vi "ADI_IMU_ADIS16470_Open.vi"(5 "Calibrate On Open":bool=TRUE, 7 "Calibration Time (s)":dbl=3.0, 8 "error in":errorcluster, 10 "Yaw Axis":enum16{"X", "Y", "Z"}(ring)=enum."Z", 11 "SPI Chip Select":T2=enum."SPI MXP") -> (0 "error out":errorcluster, 2 "Offset Compensated Data Out":dbl[](array[numeric]), 3 "ADI IMU DevRef Out":T1={"DevStatus"={"status"=FALSE, "code"=0, "source"=""}, "Handle"=0, "SPI Bus"=enum."SPI On-Board, CS0", "Device Found"=FALSE, "Device Ready"=FALSE, "Yaw Axis"=enum."Z", "Serial"=0, "Bytes Per Sample"=0, "Calibrate On Open?"=FALSE})   [LabVIEW 2017, in "ADIS16470_IMU.lvlib"]
doc: "Initiates communication between an Analog Devices MXP IMU and the RoboRIO."
uses:
  ADIS16470_IMU.lvlib
  <vilib>/Rock Robotics/SystemInterfaces/spilib/spi_bus.ctl
  ADI_IMU_ADIS16470_IMUDevRef.ctl
  <vilib>/Rock Robotics/WPI/SPI/WPI_SPIMode.ctl
  <vilib>/Rock Robotics/SystemInterfaces/DIO/FPGA_DIOChannel.ctl
  ADI_IMU_ADIS16470_Registers.ctl
  <vilib>/Rock Robotics/SystemInterfaces/NetworkCommunication/NetComm_UsageReport_ResourceType.ctl
  <vilib>/Rock Robotics/WPI/Counter/WPI_CounterDigitalInputToDigitalSource.vi
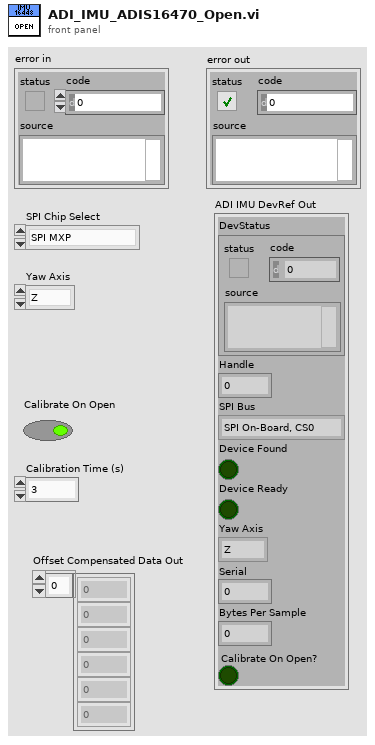
[diagram p1: front panel]
types:
  T1 = typedef "ADIS16470_IMU.lvlib/ADI_IMU_ADIS16470_IMUDevRef.ctl" = cluster{"DevStatus":errorcluster, "Handle":i32, "SPI Bus":T2, "Device Found":bool, "Device Ready":bool, "Yaw Axis":enum16{"X", "Y", "Z"}, "Serial":u16, "Bytes Per Sample":u16, "Calibrate On Open?":bool}
  T2 = typedef "spi_bus.ctl" = enum16{"SPI On-Board, CS0", "SPI On-Board, CS1", "SPI On-Board, CS2", "SPI On-Board, CS3", "SPI MXP", "Invalid"}
  T3 = typedef "FPGA_DIOChannel.ctl" = enum8{"DIO 0", "DIO 1", "DIO 2", "DIO 3", "DIO 4", "DIO 5", "DIO 6", "DIO 7", "DIO 8", "DIO 9", "DIO MXP 0", "DIO MXP 1", "DIO MXP 2", "DIO MXP 3", "DIO MXP 4", "DIO MXP 5", "DIO MXP 6", "DIO MXP 7", "DIO MXP 8", "DIO MXP 9", "DIO MXP 10", "DIO MXP 11", "DIO MXP 12", "DIO MXP 13", "DIO MXP 14", "DIO MXP 15", "SPI Port CS1", "SPI Port CS2", "SPI Port CS3", "SPI Port MISO", "SPI Port MOSI", "Invalid"}
  T4 = typedef "WPI_SPIMode.ctl" = enum16{"Mode 0 (Clk Idle Low,Sample on Leading)", "Mode 1 (Clk Idle Low,Sample on Trailing)", "Mode 2 (Clk Idle High,Sample on Leading)", "Mode 3 (Clk Idle High,Sample on Trailing)"}
  T5 = typedef "NetComm_UsageReport_ResourceType.ctl" = enum8{"Controller", "Module", "Language", "CANPlugin", "Accelerometer", "ADXL345", "AnalogChannel", "AnalogTrigger", "AnalogTriggerOutput", "CANJaguar", "Compressor", "Counter", "Dashboard", "DigitalInput", "DigitalOutput", "DriverStationCIO", "DriverStationEIO", "DriverStationLCD", "Encoder", "GearTooth", "Gyro", "I2C", "Framework", "Jaguar", "Joystick", "Kinect", "KinectStick", "PIDController", "Preferences", "PWM", "Relay", "RobotDrive", "SerialPort", "Servo", "Solenoid", "SPI", "Task", "Ultrasonic", "Victor", "Button", "Command", "AxisCamera", "PCVideoServer", "SmartDashboard", "Talon", "HiTechnicColorSensor", "HiTechnicAccel", "HiTechnicCompass", "SRF08", "AnalogOutput", "Victor SP", "Talon SRX", "CAN Talon SRX", "ADXL362 Accel", "ADXRS450 Gyro", "Rev SPARK", "Mindsensors SD540", "Digital Filter", "ADIS16448", "PDP", "PCM", "PigeonIMU", "Nidec Brushless", "CTRE CANifier", "CTRE Future 0", "CTRE Future 1", "CTRE Future 2", "CTRE Future 3", "CTRE Future 4", "CTRE Future 5", "CTRE Future 6"}
  T6 = typedef "ADIS16470_IMU.lvlib/ADI_IMU_ADIS16470_Registers.ctl" = u8
  T7 = typedef "WPI_DigitalOutputDevRef.ctl" = cluster{"DIO Channel":T3, "DevStatus":errorcluster}
  T8 = typedef "WPI_DigitalInputDevRef.ctl" = cluster{"DevStatus":errorcluster, "DIO Channel":T3}
  T9 = typedef "WPI_SPIDevRef.ctl" = cluster{"DevStatus":errorcluster, "Handle":i32, "SPI Bus":T2}
  T10 = typedef "FPGA_CounterEncoderSourceConvertionLVSourceType.ctl" = cluster{"DevStatus":errorcluster, "AnalogTriggerMode?":bool, "DigitalMode":cluster{"DIO Channel":T11}, "AnalogTriggerMode":cluster{"AnalogTriggerIndex":T12, "OutputType":T13}}
  T11 = typedef "FPGA_DIODigitalSourceChannel.ctl" = enum8{"DIO 0", "DIO 1", "DIO 2", "DIO 3", "DIO 4", "DIO 5", "DIO 6", "DIO 7", "DIO 8", "DIO 9", "DIO MXP 0", "DIO MXP 1", "DIO MXP 2", "DIO MXP 3", "DIO MXP 4", "DIO MXP 5", "DIO MXP 6", "DIO MXP 7", "DIO MXP 8", "DIO MXP 9", "DIO MXP 10", "DIO MXP 11", "DIO MXP 12", "DIO MXP 13", "DIO MXP 14", "DIO MXP 15", "SPI Port CS1", "SPI Port CS2", "SPI Port CS3", "SPI Port MISO", "SPI Port MOSI", "Disabled"}
  T12 = typedef "FPGA_AnalogTriggerIndex.ctl" = enum8{"Trig 0", "Trig 1", "Trig 2", "Trig 3", "Trig 4", "Trig 5", "Trig 6", "Trig 7", "Invalid"}
  T13 = typedef "FPGA_AnalogTriggerOutType.ctl" = enum16{"InWindow", "TriggerState", "Rising", "Falling"}
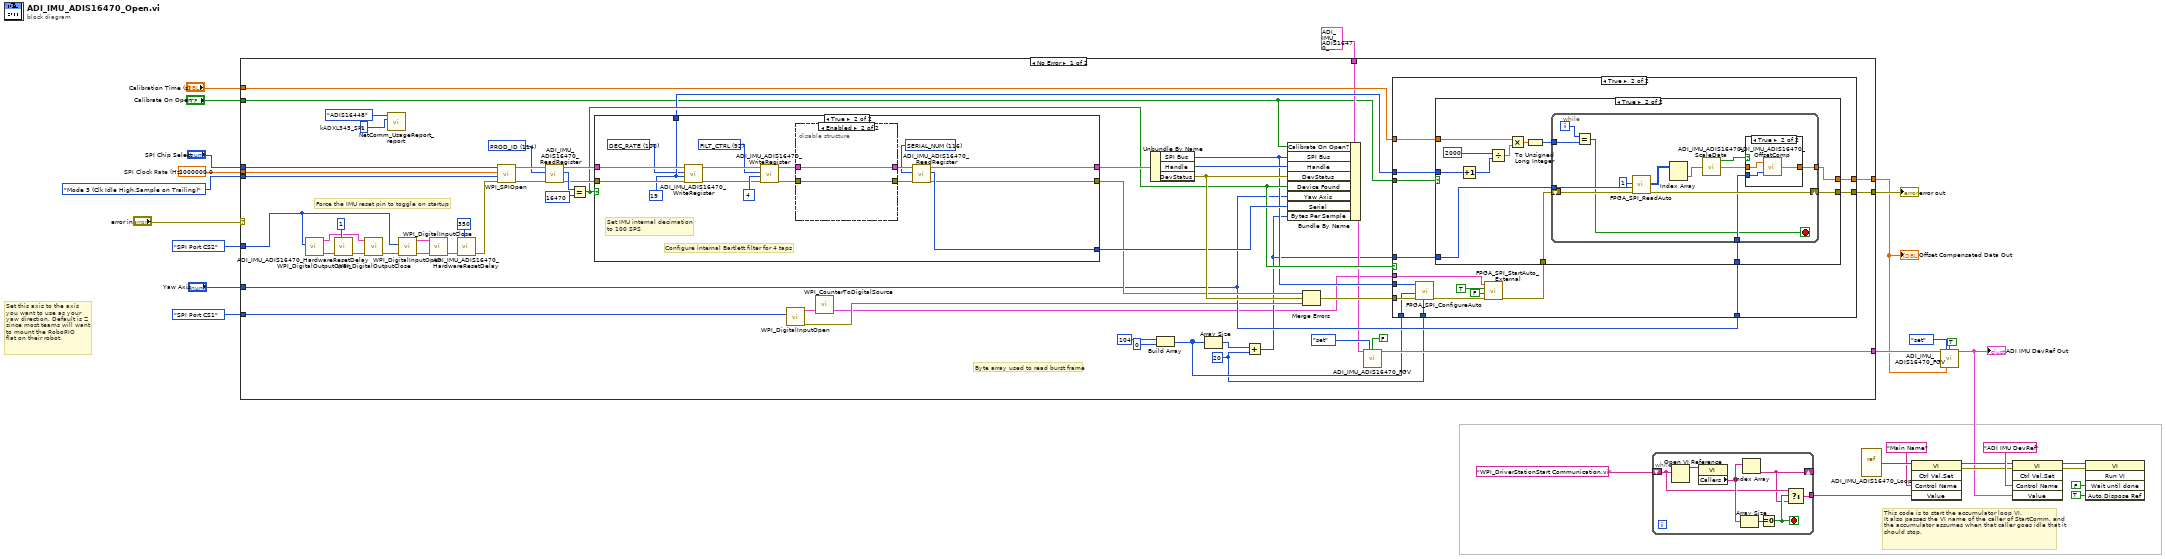
[diagram p0: block diagram]
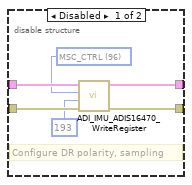
[diagram p6: hidden frame]
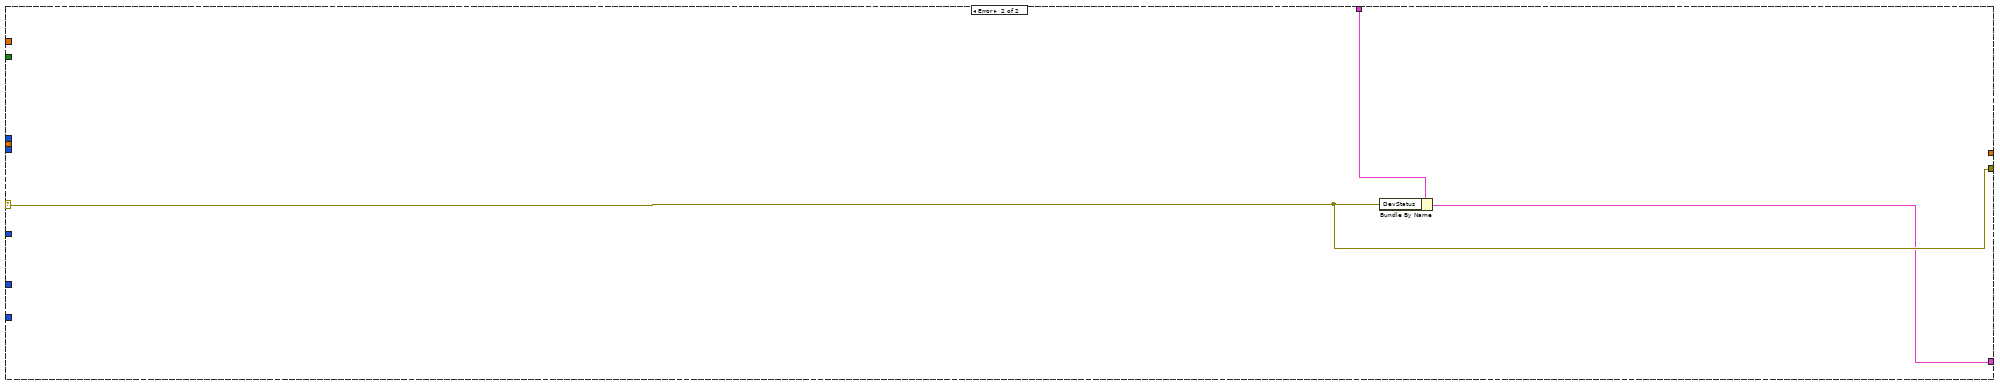
[diagram p7: hidden frame]
diagram:
  w27 = 1000000.0  # SPI Clock Rate (Hz)
  # "This code is to start the accumulator loop VI.\nIt also passes the VI name of the caller of StartComm, and the accumulator assumes when that caller goes idle that it should stop."
  # "Set this axis to the axis\nyou want to use as your\nyaw direction. Default is Z\nsince most teams will want \nto mount the RoboRIO\nflat on their robot."
  n1 = case shown="No Error" "error in" {
    selector: "error in" -> [_ w154]
    tunnel: w27 -> [w79 _]
    tunnel: WPI_SPIMode."Mode 3 (Clk Idle High,Sample on Trailing)" ("Mode (3)") -> [w78 _]
    tunnel: "SPI Chip Select" -> [w77 _]
    tunnel: FPGA_DIOChannel."SPI Port CS1" ("DIO Channel") -> [w57 _]
    tunnel: "Yaw Axis" -> [w54 _]
    tunnel: FPGA_DIOChannel."SPI Port CS2" ("DIO Channel") -> [w76 _]
    tunnel: "Calibrate On Open" -> [w33 _]
    tunnel: "Calibration Time (s)" -> [w55 _]
    tunnel: T1 {"DevStatus"={"status"=FALSE, "code"=0, "source"=""}, "Handle"=0, "SPI Bus"=enum."SPI On-Board, CS0", "Device Found"=FALSE, "Device Ready"=FALSE, "Yaw Axis"=enum."Z", "Serial"=0, "Bytes Per Sample"=0, "Calibrate On Open?"=FALSE} ("SimpleGyroDevRef 2") -> [w53 w155]
    tunnel: [w52 w154] -> w6
    tunnel: [w48 w153] -> w3
    tunnel: [w47 _] -> w2
    frame No Error {
      w30 = 20 ("dimension size")
      w71 = u8 1  # kADXL345_SPI
      w67 = T6 114 items=["DIAG_STAT"=2, "X_GYRO"=6, "Y_GYRO"=10, "Z_GYRO"=14, "X_ACCEL"=18, "Y_ACCEL"=22, "Z_ACCEL"=26, "TEMP"=28, "TIME_STAMP"=30, "FILT_CTRL"=92, "MSC_CTRL"=96, "DEC_RATE"=100, "NULL_CFG"=102, "GLOB_CMD"=104, "PROD_ID"=114, "SERIAL_NUM"=116] ("ADIS16448 Register")
      # "Byte array used to read burst frame"
      # "Force the IMU reset pin to toggle on startup"
      n2 = call <vilib>:"WPI_DigitalOutputOpen.vi"("DIO Channel"=w76) -> ("error out"=w44:errorcluster, "DigitalOutputDevRef"=w38:T7)  [unwired: 9 in]
      n3 = call "ADI_IMU_ADIS16470_HardwareResetDelay.vi"("Delay (ms)"=u32 1, "error in"=w44) -> ("error out"=w45:errorcluster)  [unwired: 9 in]
      n4 = call <vilib>:"WPI_DigitalOutputClose.vi"("error in (no error)"=w45, "DigitalOutputDevRef"=w38) -> ("error out"=w43:errorcluster)  [unwired: 9 in]
      n5 = call <vilib>:"NetComm_UsageReport_report.vi"("Instance Number"=w71, "Resource Type"=NetComm_UsageReport_ResourceType."ADIS16448") -> ()  [unwired: 10 in]
      n6 = call <vilib>:"WPI_DigitalInputOpen.vi"("error in (no error)"=w43, "DIO Channel"=w76) -> ("error out"=w42:errorcluster, "DigitalInputDevRef"=w41:T8)  [unwired: 8 in]
      n7 = call <vilib>:"WPI_DigitalInputClose.vi"("error in (no error)"=w42, "DigitalInputDevRef"=w41) -> ("error out"=w40:errorcluster)  [unwired: 9 in]
      n8 = call "ADI_IMU_ADIS16470_HardwareResetDelay.vi"("Delay (ms)"=u32 350, "error in"=w40) -> ("error out"=w72:errorcluster)  [unwired: 9 in]
      n9 = call <vilib>:"WPI_SPIOpen.vi"("error in"=w72, "Mode (3)"=w78, "Clock Rate (Hz)"=w79, "SPI Bus"=w77) -> ("error out"=w68:errorcluster, "SPIDevRef"=w69:T9)  [unwired: 6 in]
      n10 = call "ADI_IMU_ADIS16470_ReadRegister.vi"("error in (no error)"=w68, "ADIS16448 Register"=w67, "SPIDevRef in"=w69) -> ("error out"=w63:errorcluster, "Register Value"=w66:u16, "SPIDevRef out"=w64:T9)  [unwired: 6 in]
      n11 = Equal?(x=w66, y=u16 16470) -> (x = y?=w59:bool)
      n12 = case shown="True" w59 {
        tunnel: [_ w143] -> w73
        tunnel: [w128 w130] -> w62
        tunnel: [w127 w129] -> w61
        tunnel: w64 -> [w128 w136]
        tunnel: w63 -> [w127 w135]
        tunnel: [_ w134] -> w56
        frame False {
        }
        frame True {
          w131 = T6 116 items=["DIAG_STAT"=2, "X_GYRO"=6, "Y_GYRO"=10, "Z_GYRO"=14, "X_ACCEL"=18, "Y_ACCEL"=22, "Z_ACCEL"=26, "TEMP"=28, "TIME_STAMP"=30, "FILT_CTRL"=92, "MSC_CTRL"=96, "DEC_RATE"=100, "NULL_CFG"=102, "GLOB_CMD"=104, "PROD_ID"=114, "SERIAL_NUM"=116] ("ADIS16448 Register")
          w132 = T6 92 items=["DIAG_STAT"=2, "X_GYRO"=6, "Y_GYRO"=10, "Z_GYRO"=14, "X_ACCEL"=18, "Y_ACCEL"=22, "Z_ACCEL"=26, "TEMP"=28, "TIME_STAMP"=30, "FILT_CTRL"=92, "MSC_CTRL"=96, "DEC_RATE"=100, "NULL_CFG"=102, "GLOB_CMD"=104, "PROD_ID"=114, "SERIAL_NUM"=116] ("ADIS16448 Register")
          w133 = T6 100 items=["DIAG_STAT"=2, "X_GYRO"=6, "Y_GYRO"=10, "Z_GYRO"=14, "X_ACCEL"=18, "Y_ACCEL"=22, "Z_ACCEL"=26, "TEMP"=28, "TIME_STAMP"=30, "FILT_CTRL"=92, "MSC_CTRL"=96, "DEC_RATE"=100, "NULL_CFG"=102, "GLOB_CMD"=104, "PROD_ID"=114, "SERIAL_NUM"=116] ("ADIS16448 Register")
          w134 = u16 19 ("Data")
          # "Configure internal Bartlett filter for 4 taps"
          # "Set IMU internal decimation\nto 100 SPS"
          n13 = call "ADI_IMU_ADIS16470_WriteRegister.vi"("error in (no error)"=w135, "Data"=w134, "ADIS16448 Register"=w133, "SPIDevRef in"=w136) -> ("error out"=w141:errorcluster, "SPIDevRef out"=w142:T9)  [unwired: 6 in]
          n14 = call "ADI_IMU_ADIS16470_WriteRegister.vi"("error in (no error)"=w141, "Data"=u16 4, "ADIS16448 Register"=w132, "SPIDevRef in"=w142) -> ("error out"=w139:errorcluster, "SPIDevRef out"=w140:T9)  [unwired: 6 in]
          n15 = disable-structure shown="Enabled" {
            disable-tunnel: w140 -> [w150 w152]
            disable-tunnel: w139 -> [w149 w151]
            disable-tunnel: [w148 w152] -> w138
            disable-tunnel: [w147 w151] -> w137
            frame Disabled {
              w145 = T6 96 items=["DIAG_STAT"=2, "X_GYRO"=6, "Y_GYRO"=10, "Z_GYRO"=14, "X_ACCEL"=18, "Y_ACCEL"=22, "Z_ACCEL"=26, "TEMP"=28, "TIME_STAMP"=30, "FILT_CTRL"=92, "MSC_CTRL"=96, "DEC_RATE"=100, "NULL_CFG"=102, "GLOB_CMD"=104, "PROD_ID"=114, "SERIAL_NUM"=116] ("ADIS16448 Register")
              # "Configure DR polarity, sampling"
              n16 = call "ADI_IMU_ADIS16470_WriteRegister.vi"("error in (no error)"=w149, "Data"=u16 193, "ADIS16448 Register"=w145, "SPIDevRef in"=w150) -> ("error out"=w147:errorcluster, "SPIDevRef out"=w148:T9)  [unwired: 6 in]
            }
            frame Enabled {
            }
          }
          n17 = call "ADI_IMU_ADIS16470_ReadRegister.vi"("error in (no error)"=w137, "ADIS16448 Register"=w131, "SPIDevRef in"=w138) -> ("error out"=w129:errorcluster, "Register Value"=w143:u16, "SPIDevRef out"=w130:T9)  [unwired: 6 in]
        }
      }
      n18 = call <vilib>:"WPI_DigitalInputOpen.vi"("DIO Channel"=w57) -> ("error out"=w37:errorcluster, "DigitalInputDevRef"=w28:T8)  [unwired: 9 in]
      n19 = call-poly <vilib>:"WPI_CounterToDigitalSource.vi"("DigitalInputDevRef"=w28) -> ("Digital Source"=w29:T10)  [unwired: 6 in]
      n20 = Unbundle By Name(w62) -> ("SPI Bus"=w58:T2, "Handle"=w75:i32, "DevStatus"=w74:errorcluster)
      n21 = Build Array(u8 104 ("hi"), u8 0 ("element")) -> (w34:u8[])
      n22 = Array Size(array=w34) -> (size(s)=w32:i32)
      n23 = Add(x=w32, y=w30) -> (x+y=w31:i32)
      n24 = Bundle By Name(cluster=w53, "Calibrate On Open?"=w33, "SPI Bus"=w58, "Handle"=w75, "DevStatus"=w74, "Device Found"=w59, "Yaw Axis"=w54, "Serial"=w73, "Bytes Per Sample"=w31) -> (w49:T1)
      n25 = Merge Errors(w61, w74, w37) -> (w60:errorcluster)
      n26 = call "ADI_IMU_ADIS16470_FGV.vi"("ADI IMU DevRef"=w49, "Operation"=enum16{"set", "get", "set reset"}."set", "Sensor Ready?"=FALSE) -> ("ADI IMU DevRef Out"=w48:T1)  [unwired: 7 in, 5 out]
      n27 = case shown="True" w59 {
        tunnel: w60 -> [w80 w96]
        tunnel: w58 -> [_ w95]
        tunnel: w34 -> [_ w83]
        tunnel: w29 -> [_ w91]
        tunnel: w33 -> [_ w90]
        tunnel: w56 -> [_ w88]
        tunnel: w55 -> [_ w87]
        tunnel: [_ w86] -> w47
        tunnel: w54 -> [_ w85]
        tunnel: [w80 w84] -> w52
        tunnel: w31 -> [_ w82]
        tunnel: w30 -> [_ w81]
        frame False {
        }
        frame True {
          n28 = call <vilib>:"FPGA_SPI_ConfigureAuto.vi"("SPI Auto Zero Byte Count"=w81, "error in"=w96, "SPI Auto TX Byte Array"=w83, "SPI Bus"=w95) -> ("error out"=w94:errorcluster)  [unwired: 7 in]
          n29 = call <vilib>:"FPGA_SPI_StartAuto_External.vi"("error in (no error)"=w94, "Falling Edge"=FALSE, "Rising Edge"=TRUE, "Source"=w91) -> ("error out"=w89:errorcluster)  [unwired: 7 in]
          n30 = case shown="True" w90 {
            tunnel: w89 -> [w97 w109]
            tunnel: w88 -> [_ w99]
            tunnel: w87 -> [_ w106]
            tunnel: [_ w104] -> w86
            tunnel: w85 -> [_ w105]
            tunnel: [w97 w103] -> w84
            tunnel: w82 -> [_ w101]
            frame False {
            }
            frame True {
              n31 = Increment(x=w99) -> (x+1=w98:u16)
              n32 = Divide(x=2000, y=w98) -> (x/y=w108:dbl)
              n33 = Multiply(x=w106, y=w108) -> (x*y=w107:dbl)
              n34 = To Unsigned Long Integer(number=w107) -> (unsigned 32bit integer=w102:u32)
              n35 = while {
                shift-right: [w121] -> w103
                shift-left: w109 -> [w122]
                tunnel: w105 -> [w120]
                tunnel: [w119] -> w104
                tunnel: w101 -> [w117]
                tunnel: w102 -> [w114]
                i -> [w115]
                stop <- w113 stop-if-true
                n36 = Equal?(x=w115, y=w114) -> (x = y?=w113:bool)
                n37 = call <vilib>:"FPGA_SPI_ReadAuto.vi"("error in (no error)"=w122, "Bytes per Sample"=w117, "Samples to Read"=u32 1) -> ("error out"=w121:errorcluster, "Data"=w112:u8[][])  [unwired: 7 in]
                n38 = Index Array(array=w112) -> (element=w111:u8[])  [unwired: 2 in]
                n39 = call "ADI_IMU_ADIS16470_ScaleData.vi"("Received Data"=w111) -> ("Data Array"=w118:dbl[], "Data Good?"=w110:bool)  [unwired: 3 in]
                n40 = case shown="True" w110 {
                  tunnel: w120 -> [_ w126]
                  tunnel: [w123 w125] -> w119
                  tunnel: w118 -> [w123 w124]
                  frame False {
                  }
                  frame True {
                    n41 = call "ADI_IMU_ADIS16470_OffsetComp.vi"("Yaw Axis"=w126, "Raw Data"=w124) -> ("Offset Compensated Data"=w125:dbl[])
                  }
                }
              }
            }
          }
        }
      }
    }
    frame Error {
      n42 = Bundle By Name(cluster=w155, "DevStatus"=w154) -> (w153:T1)
    }
  }
  "error out" <- w6
  "Offset Compensated Data Out" <- w2
  n43 = while {
    shift-right: [w157] -> _
    shift-left: "WPI_DriverStationStart Communication.vi" -> [w158]
    tunnel: [w156] -> w12
    stop <- w159 stop-if-true
    n44 = Open VI Reference(vi path=w158) -> (vi reference=w162:refnum<vi>)  [unwired: 1 in, 5 out]
    n45 = property class="VI"(reference=w162) -> ("Callers"=w160:string[])  [unwired: 1 in, 2 out]
    n46 = Array Size(array=w160) -> (size(s)=w161:i32)
    n47 = Index Array(array=w160) -> (element=w157:string)  [unwired: 1 in]
    n48 = Equal To 0?(x=w161) -> (x = 0?=w159:bool)
    n49 = Select(t=w158, s=w159, f=w157) -> (s? t:f=w156:string)
  }
  n50 = vi-ref "ADI_IMU_ADIS16470_Loop.vi"() -> (w14:refnum<vi>)
  n51 = invoke class="VI" method="Ctrl Val.Set"(reference=w14, "Control Name"="Main Name", "Value"=w12) -> (reference out=w11:refnum<vi>, error out=w16:errorcluster)  [unwired: 2 in, 3 out]
  n52 = call "ADI_IMU_ADIS16470_FGV.vi"("ADI IMU DevRef"=w3, "Operation"=enum16{"set", "get", "set reset"}."set", "Sensor Ready?"=TRUE, "Offset Compensated Data"=w2) -> ("ADI IMU DevRef Out"=w1:T1)  [unwired: 6 in, 5 out]
  "ADI IMU DevRef Out" <- w1
  n53 = invoke class="VI" method="Ctrl Val.Set"(reference=w11, error in=w16, "Control Name"="ADI IMU DevRef", "Value"=w1) -> (reference out=w21:refnum<vi>, error out=w17:errorcluster)  [unwired: 1 in, 3 out]
  n54 = invoke class="VI" method="Run VI"(reference=w21, error in=w17, "Wait until done"=FALSE ("Wait Until Done"), "Auto Dispose Ref"=TRUE ("Auto Dispose Reference")) -> ()  [unwired: 1 in, 5 out]
